vi "Connect.vi"(8 "error in (no error)":errorcluster, 10 "Channel(s)":string, 11 "NI Switch in":refnum<class "NI Switch.lvclass">) -> (0 "error out":errorcluster, 3 "NI Switch out":refnum<class "NI Switch.lvclass">)   [LabVIEW 2025, in "Switch.lvlib" / "NI Switch.lvclass"]
uses:
  NI Switch.lvclass
  NI Switch.lvclass/NI Switch.ctl
  <instrlib>/niSwitch/niSwitch.llb/niSwitch Connect Channels (Multiple).vi
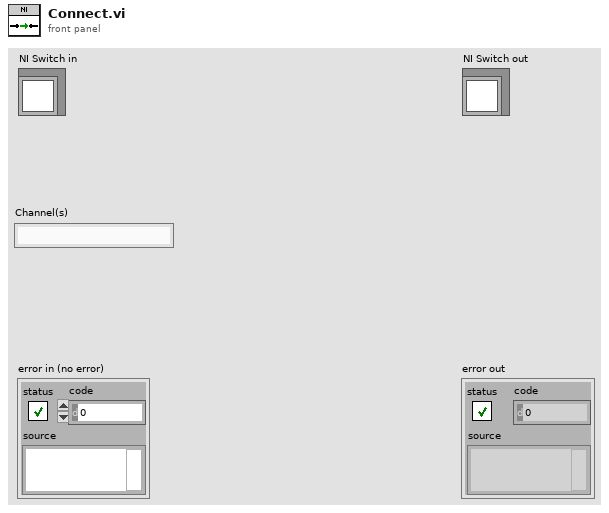
[diagram p1: front panel]
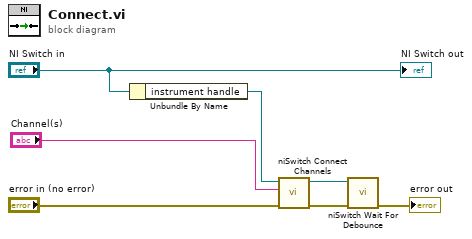
[diagram p0: block diagram]
diagram:
  n1 = Unbundle By Name("NI Switch in") -> ("instrument handle"=w2:refnum<k15>)
  n2 = call-poly <instrlib>:"niSwitch Connect Channels.vi"("error in (no error)"="error in (no error)", "connection list"="Channel(s)", "instrument handle"=w2) -> ("error out"=w6:errorcluster, "instrument handle out"=w7:refnum<k15>)  [unwired: 7 in]
  n3 = call <instrlib>:"niSwitch Wait For Debounce.vi"("error in (no error)"=w6, "instrument handle"=w7) -> ("error out"=→"error out":errorcluster)  [unwired: 8 in, 1 out]
  "NI Switch out" <- "NI Switch in"
